vi "GetFileTree.vi"(6 "patterns":string[](array[string])=["*.py"], 7 "Font Color":u32(colorbox)=16713728, 8 "StartRow":u32, 9 "Tree":refnum<vi>, 10 "Open?":bool, 11 "Base Path":path) -> (0 "NumRows":u32, 2 "File list":path[](array[path]))   [LabVIEW 2022 SP3]
panel:
  in  "Tree":string(tree)
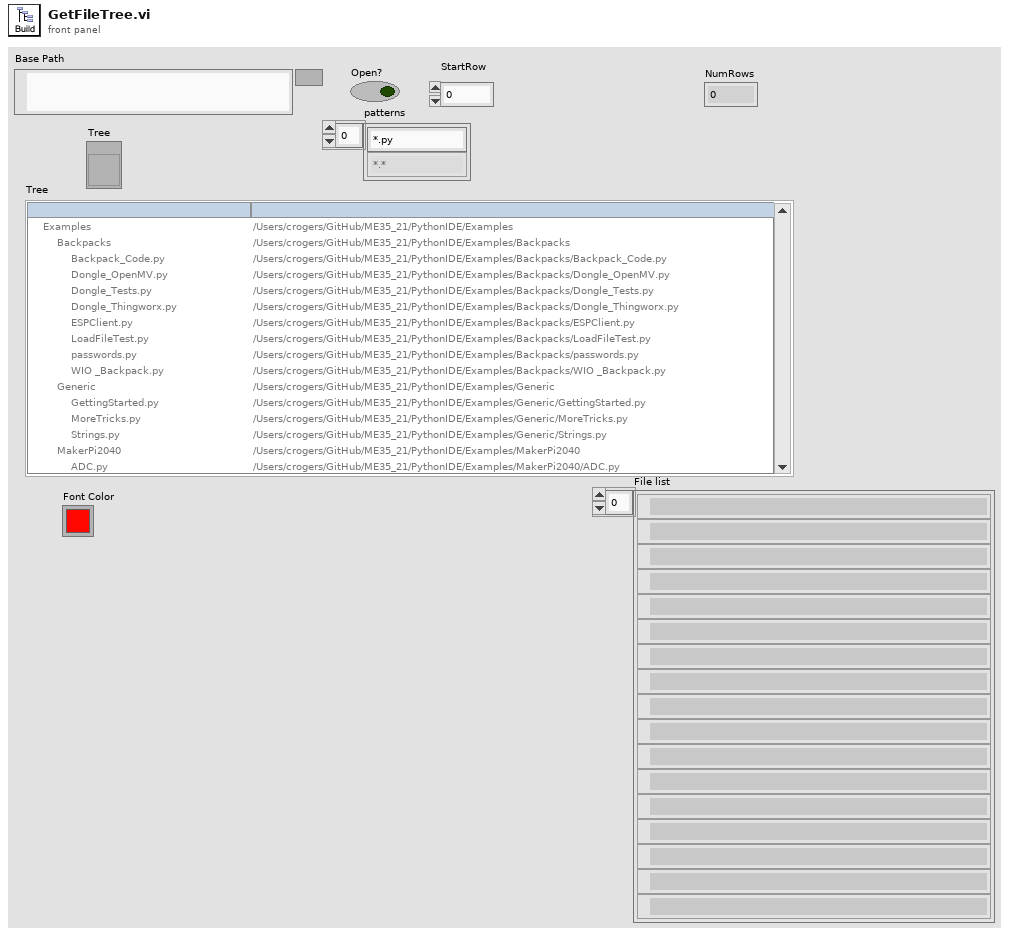
[diagram p1: front panel]
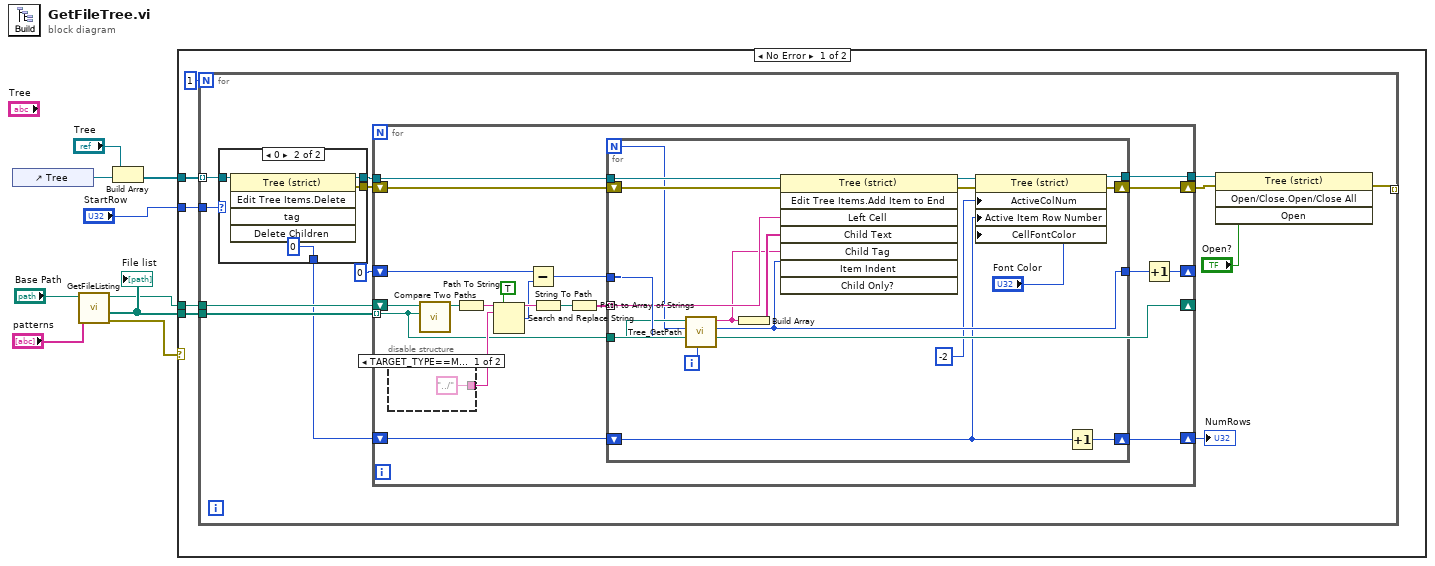
[diagram p0: block diagram]
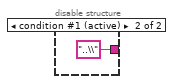
[diagram p3: hidden frame]
diagram:
  n1 = control-ref of="Tree"() -> (w7:refnum<vi>)
  n2 = call "GetFileListing.vi"("patterns"="patterns", "Base Path"="Base Path") -> ("error out"=w9:errorcluster, "Files"=w5:path[], "Base"=w2:path)  [unwired: 7 in]
  "File list" <- w5
  n3 = Build Array("Tree", w7) -> (w6:refnum<vi>[])
  n4 = case shown="No Error" w9 {
    tunnel: w6 -> [w14 _]
    tunnel: w5 -> [w13 _]
    tunnel: w2 -> [w12 _]
    tunnel: "StartRow" -> [w11 _]
    frame No Error {
      n5 = for {
        N: 1 -> [_]
        tunnel: w14 -> [w27] mode=indexing
        tunnel: w13 -> [w25]
        tunnel: w12 -> [w24]
        tunnel: [w18] -> _ mode=indexing
        tunnel: w11 -> [w17]
        n6 = case shown="0" w17 {
          selector: w17 -> [w28 _]
          tunnel: w27 -> [w29 w33]
          tunnel: [w29 w32] -> w23
          tunnel: [_ w31] -> w20
          tunnel: [w28 0] -> w16
          frame Default {
          }
          frame 0 {
            n7 = invoke on="Invoke Node" class="Tree (strict)" method="Edit Tree Items.Delete"(reference=w33) -> (reference out=w32:refnum<vi>, error out=w31:errorcluster)  [unwired: 4 in, 3 out]
          }
        }
        n8 = for {
          tunnel: w25 -> [w34] mode=indexing
          shift-right: [w34] -> _
          shift-left: w24 -> [w53]
          shift-right: [w41] -> _
          shift-left: 0 -> [w43]
          tunnel: w23 -> [w40]
          tunnel: [w39] -> w21
          shift-right: [w37] -> w19
          shift-left: w20 -> [w38]
          shift-right: [w35] -> w15
          shift-left: w16 -> [w36]
          n9 = disable-structure shown="TARGET_TYPE==Mac" {
            disable-tunnel: ["../" ("search string") "..\\" ("search string")] -> w51
            frame condition #0 {
            }
            frame condition #1 (active) {
            }
          }
          n10 = call <vilib>:"Compare Two Paths.vi"("Path 2"=w34, "Path 1"=w53) -> ("Relative Path from 1 to 2"=w45:path)  [unwired: 6 in, 3 out]
          n11 = Path To String(path=w45) -> (string=w52:string)
          n12 = Search and Replace String(replace all?=TRUE ("replace all? (F)"), input string=w52, search string=w51) -> (result string=w49:string, number of replacements=w46:i32)  [unwired: 5 in, 2 out]
          n13 = Subtract(x=w43, y=w46) -> (x-y=w44:i32)
          n14 = String To Path(string=w49) -> (path=w48:path)
          n15 = Path to Array of Strings(0:w48) -> (2:w47:string[])  [unwired: 1 out]
          n16 = for {
            N -> [w57]
            tunnel: w47 -> [w67] mode=indexing
            tunnel: w44 -> [w71]
            tunnel: [w70] -> w42
            tunnel: w40 -> [w64]
            tunnel: [w64] -> w39
            shift-right: [w59] -> w37
            shift-left: w38 -> [w68]
            shift-right: [w65] -> w35
            shift-left: w36 -> [w62]
            tunnel: w34 -> [w58]
            i -> [w56]
            n17 = call "Tree_GetPath.vi"("i"=w56, "level"=w71, "# Folders"=w57, "Path"=w58) -> ("indent"=w70:i32, "path"=w66:string)  [unwired: 6 in]
            n18 = Build Array(w66) -> (w69:string[])
            n19 = invoke on="Invoke Node" class="Tree (strict)" method="Edit Tree Items.Add Item to End"(reference=w64, error in=w68, "Left Cell"=w67, "Child Text"=w69, "Child Tag"=w66, "Item Indent"=w70) -> (error out=w60:errorcluster)  [unwired: 2 in, 7 out]
            n20 = property class="Tree (strict)"(reference=w64, error in=w60, "ActiveColNum"=-2 ("Active Cell:Active Column Number"), "Active Item Row Number"=w62, "CellFontColor"="Font Color") -> (error out=w59:errorcluster)  [unwired: 1 out]
            n21 = Increment(x=w62) -> (x+1=w65:u32)
          }
          n22 = Increment(x=w42) -> (x+1=w41:i32)
        }
        "NumRows" <- w15
        n23 = invoke on="Invoke Node" class="Tree (strict)" method="Open/Close.Open/Close All"(reference=w21, error in=w19, "Open"="Open?") -> (error out=w18:errorcluster)  [unwired: 1 in, 3 out]
      }
    }
    frame Error {
    }
  }
